vi "Untitled 1.vi"() -> ()   [LabVIEW 2016]
uses:
  <vilib>/DNP3/DNP3_Common/Create Channel (IP Networking).vi
  <vilib>/DNP3/DNP3_Outstation.lvlib
  <vilib>/DNP3/DNP3_Common.lvlib
panel:
  out "error out":errorcluster
  out "OS_Network_Settings_Initial":T1
  out "DNP3 DataMap_Initial":T2={"Binary Output Points"=1, "Binary Input Points"=0, "Analog Output Points"=7, "Analog Input Points"=6}
  in  "Network Settings 1":T1={"port (20000)"=18000, "Master IP"="48.26.87.212", "Master Address"=12345, "Outstation Address "=54321, " update rate"=50}
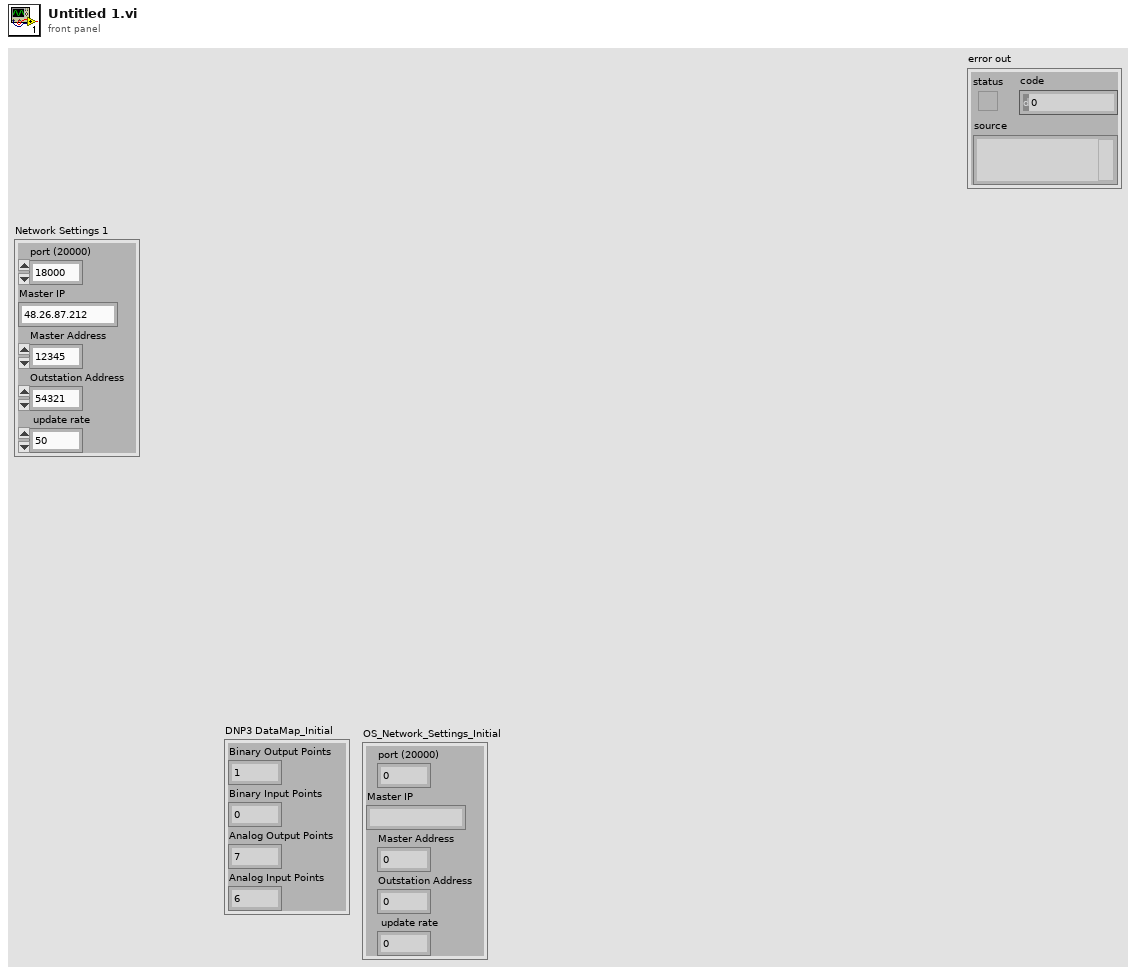
[diagram p1: front panel]
types:
  T1 = cluster{"port (20000)":u16, "Master IP":string, "Master Address":u16, "Outstation Address ":u16, " update rate":u32}
  T2 = cluster{"Binary Output Points":u16, "Binary Input Points":u16, "Analog Output Points":u16, "Analog Input Points":u16}
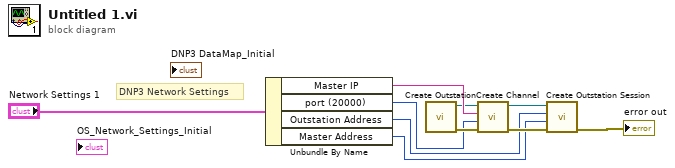
[diagram p0: block diagram]
diagram:
  # "DNP3 Network Settings"
  n1 = Unbundle By Name("Network Settings 1") -> ("Master IP"=w7:string, "port (20000)"=w6:u16, "Outstation Address"=w5:u16, "Master Address"=w4:u16)
  n2 = call <vilib>:"Create Outstation.vi"() -> ("error out"=w10:errorcluster, "DNP3 outstation out"=w3:refnum<k21>)  [unwired: 10 in]
  n3 = call-poly <vilib>:"Create Channel.vi"("error in (no error)"=w10, "port (20000)"=w6, "IP"=w7, "DNP3 outstation"=w3) -> ("error out"=w9:errorcluster, "DNP3 channel out"=w8:refnum<k21>)  [unwired: 6 in]
  n4 = call <vilib>:"Create Outstation Session.vi"("error in (no error)"=w9, "destination"=w4, "source"=w5, "DNP3 channel"=w8) -> ("error out"=→"error out":errorcluster)  [unwired: 6 in, 1 out]
